vi "Set plot legend size and pos.vi"(9 "Data In (ordered by ROI index)":T1, 11 "WaveformGraph in":T6) -> (3 "WaveformGraph out":T6)   [LabVIEW 2017]
uses:
  Typedefs/Xctrl-Waveform graph ref.ctl
  Data 1.ctl
  Typedefs/Xctrl-Data array.ctl
  Typedefs/Xcrtl-Data format definition.ctl
  Typedefs/Xctl-XY data type definition.ctl
  Typedefs/Xctrl-ROI type enum.ctl
  XGrapher.xctl
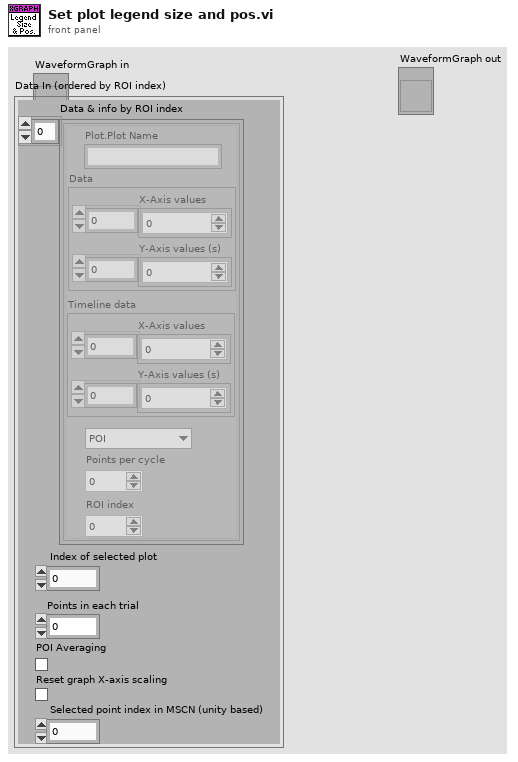
[diagram p1: front panel]
types:
  T1 = typedef "XGrapher.xctl/Data 1.ctl" = cluster{"Data & info by ROI index":T2, "Index of selected plot":u16, "Points in each trial":i32, "POI Averaging":bool, "Reset graph X-axis scaling":bool, "Selected point index in MSCN (unity based)":u16}
  T2 = typedef "Xctrl-Data array.ctl" = T3[]
  T3 = typedef "XGrapher.xctl/Xcrtl-Data format definition.ctl" = cluster{"Plot.Plot Name":string, "Data":T4, "Timeline data":T4, "Type":T5, "Points per cycle":u16, "ROI index":u16}
  T4 = typedef "XGrapher.xctl/Xctl-XY data type definition.ctl" = cluster{"X-Axis values":sgl[], "Y-Axis values (s)":sgl[]}
  T5 = typedef "Xctrl-ROI type enum.ctl" = enum16{"POI", "Mini-scan", "Group"}
  T6 = typedef "XGrapher.xctl/Xctrl-Waveform graph ref.ctl" = refnum<vi>
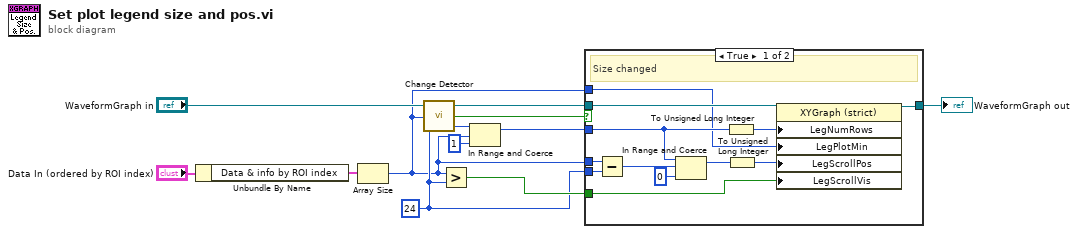
[diagram p0: block diagram]
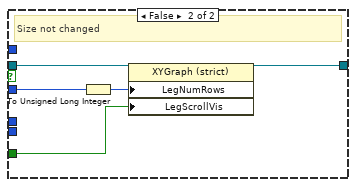
[diagram p2: hidden frame]
diagram:
  w2 = 24 ("Legend:Number of Rows")
  n1 = Unbundle By Name("Data In (ordered by ROI index)") -> ("Data & info by ROI index"=w7:T2)
  n2 = Array Size(array=w7) -> (size(s)=w1:i32)
  n3 = call <userlib>:"Change Detector.vi"("Value"=w1) -> ("Changed?"=w3:bool)
  n4 = Greater?(x=w1, y=w2) -> (0:w6:bool)
  n5 = In Range and Coerce(upper limit=w2, x=w1, lower limit=1) -> (coerced(x)=w5:i32)  [unwired: 1 out]
  n6 = case shown="True" w3 {
    tunnel: "WaveformGraph in" -> [w22 w27]
    tunnel: [w21 w26] -> w8
    tunnel: w6 -> [w20 w24]
    tunnel: w5 -> [w12 w25]
    tunnel: w2 -> [w19 _]
    tunnel: w1 -> [w16 _]
    tunnel: w1 -> [w11 _]
    frame True {
      # "Size changed"
      n7 = Subtract(x=w16, y=w19) -> (x-y=w13:i32)
      n8 = In Range and Coerce(upper limit=w12, x=w13, lower limit=0) -> (coerced(x)=w17:i32)  [unwired: 1 out]
      n9 = To Unsigned Long Integer(number=w12) -> (unsigned 32bit integer=w14:u32)
      n10 = To Unsigned Long Integer(number=w17) -> (unsigned 32bit integer=w15:u32)
      n11 = property on="Property Node" class="XYGraph (strict)"(reference=w22, "LegNumRows"=w14, "LegPlotMin"=w11, "LegScrollPos"=w15, "LegScrollVis"=w20) -> (reference out=w21:T6)  [unwired: 1 in, 1 out]
    }
    frame False {
      # "Size not changed"
      n12 = To Unsigned Long Integer(number=w25) -> (unsigned 32bit integer=w23:u32)
      n13 = property on="Property Node" class="XYGraph (strict)"(reference=w27, "LegNumRows"=w23, "LegScrollVis"=w24) -> (reference out=w26:T6)  [unwired: 1 in, 1 out]
    }
  }
  "WaveformGraph out" <- w8
